vi "Discover SSH Device.vi"(8 "error in (no error)":errorcluster, 10 "Password":string, 11 "user@host":string) -> (0 "error out":errorcluster)   [LabVIEW 2024, in "Session Scanner.lvlib"]
uses:
  Session Scanner.lvlib
  <vilib>/net/SSH/Client/OpenSSH/OpenSSH Client.lvclass
  <vilib>/net/SSH/NI_SSH.lvlib
  C:/Program Files (x86)/National Instruments/LabVIEW 2024/vi.lib/net/SSH/Client/Generic/Generic Client.lvclass
  C:/Program Files (x86)/National Instruments/LabVIEW 2024/vi.lib/net/SSH/Client/OpenSSH/OpenSSH Client.lvclass
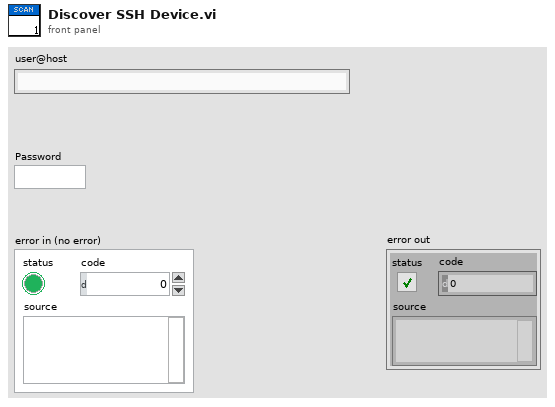
[diagram p1: front panel]
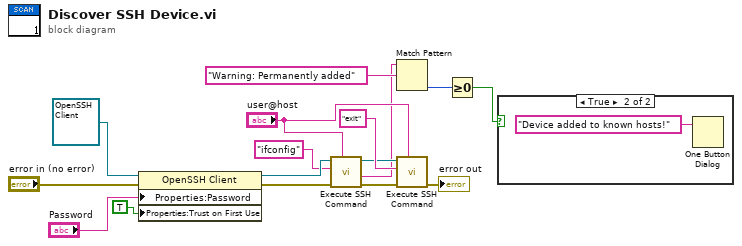
[diagram p0: block diagram]
diagram:
  n1 = property class="OpenSSH Client"(reference=refnum<class "OpenSSH Client.lvclass"> refnum ("NI_SSH.lvlib:OpenSSH Client"), error in="error in (no error)", "Properties:Password"="Password", "Properties:Trust on First Use"=TRUE ("Trust on First Use")) -> (reference out=w12:refnum<class "OpenSSH Client.lvclass">, error out=w7:errorcluster)
  n2 = call <vilib>:"Execute SSH Command.vi"("user@host"="user@host", "error in (no error)"=w7, "command line"="ifconfig", "session in"=w12) -> ("error out"=w8:errorcluster, "standard error"=w4:string, "session out"=w9:refnum<class "OpenSSH Client.lvclass">)  [unwired: 3 in, 2 out]
  n3 = Match Pattern(string=w4, regular expression="Warning: Permanently added" ("scrollbar text")) -> (offset past match=w6:i32)  [unwired: 1 in, 3 out]
  n4 = call <vilib>:"Execute SSH Command.vi"("user@host"="user@host", "error in (no error)"=w8, "command line"="exit", "session in"=w9) -> ("error out"=→"error out":errorcluster)  [unwired: 3 in, 4 out]
  n5 = Greater Or Equal To 0?(x=w6) -> (x >= 0?=w13:bool)
  n6 = case shown="True" w13 {
    frame False {
    }
    frame True {
      n7 = One Button Dialog(message="Device added to known hosts!") -> ()  [unwired: 1 in, 1 out]
    }
  }
